vi "PicoScope5000aSetEts.vi"(7 "ETS Mode":u32(ring) items=["PS5000A_ETS_OFF", "PS5000A_ETS_FAST", "PS5000A_ETS_SLOW"], 8 "error in (no error)":errorcluster, 9 "etsInterleave":i16, 10 "etsCycles":i16, 11 "handle in":i16) -> (0 "error out":errorcluster, 3 "handle out":i16, 4 "sampleTimePicoseconds":i32)   [LabVIEW 2009]
doc: "Calls SetETS"
uses:
  ps5000a.dll
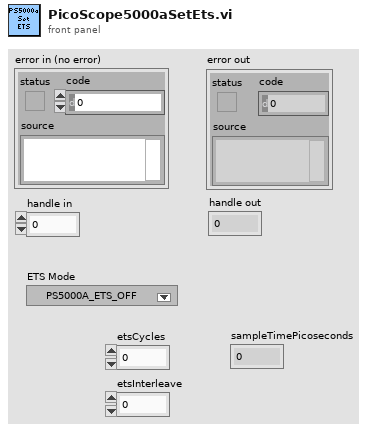
[diagram p1: front panel]
types:
  T1 = cluster{"status":bool, "code":u32, "source":string}
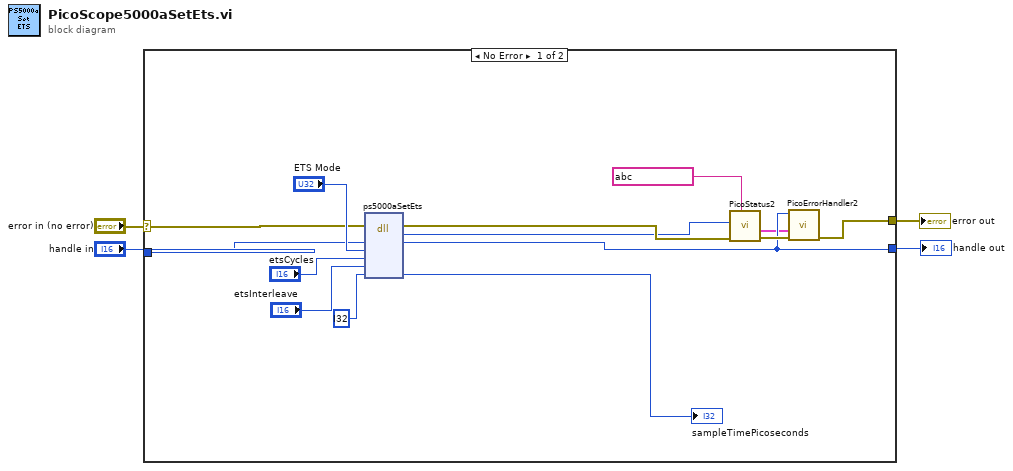
[diagram p0: block diagram]
diagram:
  n1 = case shown="No Error" "error in (no error)" {
    selector: "error in (no error)" -> [w14 w20]
    tunnel: [w17 w20] -> w2
    tunnel: "handle in" -> [w13 w19]
    tunnel: [w12 w19] -> w3
    frame #0 {
      n2 = dll-call lib="ps5000a.dll" fn="ps5000aSetEts" ("ps3000.dll:_ps3000_open_unit@0")(error in=w14, "handle"=w13, "mode"="ETS Mode", "etsCycles"="etsCycles", "etsInterleave"="etsInterleave", "sampleTimePicoseconds"=i32 ?) -> (error out=w6:errorcluster, "PICO_STATUS"=w5:u32, "handle"=w12:i16, "sampleTimePicoseconds"=→"sampleTimePicoseconds":i32)  [unwired: 5 in, 1 out]
      n3 = call "PicoStatus2.vi"("PICO source"=string ? ("source"), "Error in"=w6, "PICO STATUS"=w5) -> ("error out"=w18:errorcluster, "PICO_STATUS out"=w8:T1)  [unwired: 5 in]
      n4 = call "PicoErrorHandler2.vi"("error in (no error)"=w18, "PICO_STATUS in"=w8, "handle In"=w12) -> ("error out"=w17:errorcluster)  [unwired: 8 in]
    }
    frame #1 {
    }
  }
  "error out" <- w2
  "handle out" <- w3
